vi "ST_parse_add_pinion_response.vi"(5 "SQL_connection_reference":T1, 7 "pinion_serial":string, 8 "error_in":errorcluster, 11 "recordset_in":variant[][](array[variant])) -> (0 "error_out":errorcluster, 2 "operation_id":string, 3 "operation_status":T2)   [LabVIEW 2020]
uses:
  SQL_statuses.ctl
  <vilib>/addons/database/Connection.llb/Conn ObjectReference.ctl
  FGV/SQL_pinion_ID_buffer/FGV_SQL_pinion_ID_buffer.ctl
  <vilib>/addons/database/_DB Variant To Data/Database Variant To Data.xnode
  <vilib>/addons/database/NI_Database_API.lvlib
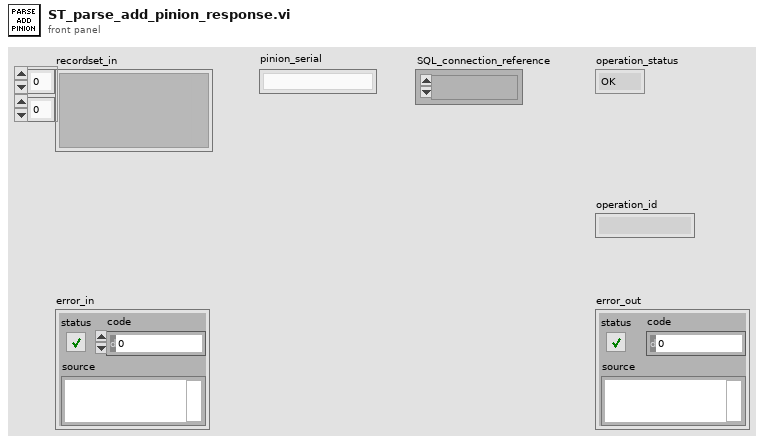
[diagram p1: front panel]
types:
  T1 = typedef "NI_Database_API.lvlib/Conn ObjectReference.ctl" = refnum<k1>
  T2 = typedef "SQL_statuses.ctl" = enum16{"OK", "PART_IN_OPERATION", "PART_DOES_NOT_EXIST", "OPERATION_DOES_NOT_EXIST", "OPERATOR_DOES_NOT_EXIST", "PART_NOT_IN_OPERATION"}
  T3 = typedef "FGV_SQL_pinion_ID_buffer.ctl" = enum16{"initialize", "buffer_pinion_ID", "buffer_pinion_ID_SQL", "get_ID_for_name"}
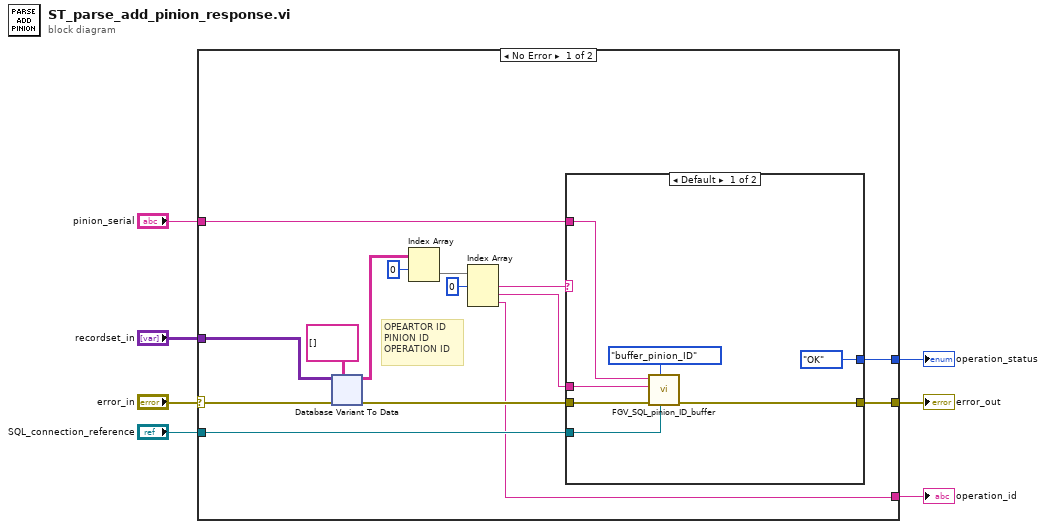
[diagram p0: block diagram]
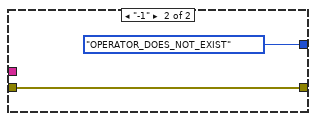
[diagram p2: hidden frame]
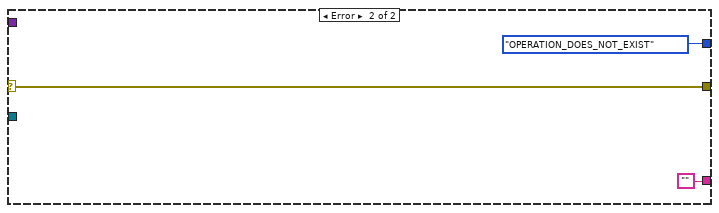
[diagram p3: hidden frame]
diagram:
  n1 = case shown="No Error" "error_in" {
    selector: "error_in" -> [w21 w78]
    tunnel: [w13 w78] -> w7
    tunnel: [w22 SQL_statuses."OPERATION_DOES_NOT_EXIST" ("SQL_statuses")] -> w5
    tunnel: "recordset_in" -> [w11 _]
    tunnel: "pinion_serial" -> [w9 _]
    tunnel: "SQL_connection_reference" -> [w12 _]
    tunnel: [w8 ""] -> w1
    frame No Error {
      # "OPEARTOR ID\nPINION ID\nOPERATION ID"
      n2 = xnode "Database Variant To Data"("database variant"=w11, "error in (no error)"=w21, "type"=string[][] []) -> ("data"=w16:string[][], "error out"=w14:errorcluster)
      n3 = Index Array(array=w16, index (row)=0) -> (element=w18:string[])  [unwired: 1 in]
      n4 = Index Array(array=w18, index #1=0 ("index")) -> (element #1=w15:string, element #2=w10:string, element #3=w8:string)  [unwired: 2 in]
      n5 = case shown="Default" w15 {
        tunnel: [SQL_statuses."OK" ("SQL_statuses") SQL_statuses."OPERATOR_DOES_NOT_EXIST" ("SQL_statuses")] -> w22
        tunnel: w14 -> [w28 w30]
        tunnel: [w27 w30] -> w13
        tunnel: w12 -> [w26 _]
        tunnel: w10 -> [w25 _]
        tunnel: w9 -> [w24 _]
        frame Default {
          n6 = call "FGV_SQL_pinion_ID_buffer.vi"("connection reference"=w26, "options"=FGV_SQL_pinion_ID_buffer."buffer_pinion_ID", "error_in"=w28, "PINION_ID"=w25, "PINION_SERIAL"=w24) -> ("error_out"=w27:errorcluster)  [unwired: 4 in, 2 out]
        }
        frame "-1" {
        }
      }
    }
    frame Error {
    }
  }
  "error_out" <- w7
  "operation_status" <- w5
  "operation_id" <- w1
